vi "nanocal frontend 18.vi"() -> ()   [LabVIEW 2018]
uses:
  nanocal/Nanocalorimetry/data/NanoCalLib.lvlibp/NanoReadings/NanoReadings_Parameters_TypeDef.ctl
  nanocal/Nanocalorimetry/data/NanoCalLib.lvlibp/NanoReadings/NanoReadings_Power.ctl
  nanocal/Nanocalorimetry/data/NanoCalLib.lvlibp/NanoReadings/NanoReadings_CandK.ctl
  nanocal/Nanocalorimetry/data/NanoCalLib.lvlibp/NanoReadings/NanoReadings_IandV.ctl
  nanocal/Nanocalorimetry/data/NanoCalLib.lvlibp/NanoReadings/NanoReadings_TdcTac.ctl
  nanocal/Nanocalorimetry/data/NanoCalLib.lvlibp/NanoReadings/NanoReadings_Phases.ctl
  nanocal/Nanocalorimetry/data/NanoCalLib.lvlibp/NanoReadings/NanoReadings_Frequencies.ctl
  nanocal/Nanocalorimetry/data/NanoCalLib.lvlibp/NanoReadings/NanoReadings_FirstHarmonic.ctl
  nanocal/Nanocalorimetry/data/NanoCalLib.lvlibp/NanoReadings/NanoReadings_Output.ctl
  nanocal/Nanocalorimetry/data/NanoCalLib.lvlibp/NanoReadings/NanoReadings_MagneticFieldEtc.ctl
  nanocal/Nanocalorimetry/data/NanoCalLib.lvlibp/NanoReadings/NanoReadings_Calibration.ctl
  nanocal/Nanocalorimetry/data/NanoCalLib.lvlibp/NanoReadings/NanoReadings_CTetc.ctl
  nanocal/Nanocalorimetry/data/NanoCalLib.lvlibp/NanoReadings/NanoReadings_2ndHarmonic.ctl
  nanocal/Nanocalorimetry/data/NanoCalLib.lvlibp/NanoReadings/NanoReadings_Resistance.ctl
  nanocal/Nanocalorimetry/data/NanoCalLib.lvlibp/NanoReadings/NanoReadings_TimeEtc.ctl
  frontend -- data type -- folder/frontend -- data type.ctl
  nanocal/Nanocalorimetry/data/NanoCalLib.lvlibp
  nanocal/Nanocalorimetry/data/NanoCalLib.lvlibp/NanoReadings/NanoReadings.lvlib
panel:
  out "Numeric":i32=90
  out "output cluster":T1
  in  "milliseconds to wait":u32=100
  in  "Stop":bool
  out "Latest data":T2 {"Time etc"."Datapoint time (s)" format="%#_7g"; "Time etc"."Datapoint index" format="%#_7g"; "Time etc"."Time (s)" format="%#_7g"; "Resistance"."Roffs (ohm)" format="%#_7g"; "Resistance"."Rr,ac (ohm)" format="%#_7g"; "Resistance"."Rs,ac (ohm)" format="%#_7g"; "Resistance"."RHr,dc (ohm)" format="%#_7g"; "Resistance"."RHs,dc (ohm)" format="%#_7g"; "Resistance"."Rr (ohm)" format="%#_7g"; "Resistance"."Rs (ohm)" format="%#_7g"; "Resistance"."RHr (ohm)" format="%#_7g"; "Resistance"."RHs (ohm)" format="%#_7g"; "IV 2nd harm"."Udiff,ac (V)" format="%#_7g"; "IV 2nd harm"."Ur,ac (V)" format="%#_7g"; "IV 2nd harm"."Us,ac (V)" format="%#_7g"; "IV 2nd harm"."Ir,ac (A)" format="%#_7g"; "IV 2nd harm"."Is,ac (A)" format="%#_7g"; "CT etc"."Tr^2 (K^2)" format="%#_7g"; "CT etc"."Ts^2 (K^2)" format="%#_7g"; "Calibration"."dTr/dt (mK/s)" format="%#_7g"; "Calibration"."dTs/dt (mK/s)" format="%#_7g"; "Output"."Hr dc out (V)" min=0.0 max=7.0707; "Output"."Hs dc out (V)" min=0.0 max=7.0707; "Output"."Hr ac out (Vrms)" min=0.0 max=7.0707; "Output"."Hs ac out (Vrms)" min=0.0 max=7.0707; "Output"."R phase (deg)" format="%#_7g"; "Output"."S phase (deg)" format="%#_7g"; "IV 1st harm"."UHr (V)" format="%#_7g"; "IV 1st harm"."IHr (A)" format="%#_7g"; "IV 1st harm"."UHs (V)" format="%#_7g"; "IV 1st harm"."IHs (A)" format="%#_7g"; "IV 1st harm"."Udiff,ac 1st (V)" format="%#_7g"; "IV 1st harm"."Ur,ac 1st (V)" format="%#_7g"; "IV 1st harm"."Us,ac 1st (V)" format="%#_7g"; "IV 1st harm"."Ir,ac 1st (A)" format="%#_7g"; "IV 1st harm"."Is,ac 1st (A)" format="%#_7g"; "f etc"."tau (s)" format="%#_7g"; "f etc"."Cos Phi" format="%#_7g"; "f etc"."Sin Phi" format="%#_7g"; "f etc"."Tan Phi S/diff" format="%#_7g"; "Phases"."Phi Udiff, raw (deg)" format="%#_7g"; "Phases"."Phi Udiff 1st (deg)" format="%#_7g"; "Phases"."Phi Ur 1st (deg)" format="%#_7g"; "Phases"."Phi Ir 1st (deg)" format="%#_7g"; "Phases"."Phi Us 1st (deg)" format="%#_7g"; "Phases"."Phi Is 1st (deg)" format="%#_7g"; "Phases"."Phi R from S,diff (deg)" format="%#_7g"; "Phases"."Phi UHr (deg)" format="%#_7g"; "Phases"."Phi IHr (deg)" format="%#_7g"; "Phases"."Phi UHs (deg)" format="%#_7g"; "Phases"."Phi IHs (deg)" format="%#_7g"; "Phases"."Phi Udiff (deg)" format="%#_7g"; "Phases"."Phi Ur (deg)" format="%#_7g"; "Phases"."Phi Ir (deg)" format="%#_7g"; "Phases"."Phi Us (deg)" format="%#_7g"; "Phases"."Phi Is (deg)" format="%#_7g"; "Tdc,Tac"."T target (K)" format="%#_7g"; "Tdc,Tac"."Tr,ac from Ts,diff,ac (K)" format="%#_7g"; "Tdc,Tac"."Tr,ac driftcorr (K)" format="%#_7g"; "Tdc,Tac"."Ts,ac driftcorr (K)" format="%#_7g"; "Tdc,Tac"."Tdiff,ac (K)" format="%#_7g"; "Tdc,Tac"."Tr,ac (K)" format="%#_7g"; "Tdc,Tac"."Ts,ac (K)" format="%#_7g"; "Tdc,Tac"."Tdiff from Udiff (K)" format="%#_7g"; "Tdc,Tac"."Tdiff from Rs,Rr" format="%#_7g"; "Tdc,Tac"."Tr (K)" format="%#_7g"; "Tdc,Tac"."Ts (K)" format="%#_7g"; "IV dc"."Ioffs dc (A)" format="%#_7g"; "IV dc"."Uoffs dc (V)" format="%#_7g"; "IV dc"."UHr dc (V)" format="%#_7g"; "IV dc"."IHr dc (A)" format="%#_7g"; "IV dc"."UHs dc (V)" format="%#_7g"; "IV dc"."IHs dc (A)" format="%#_7g"; "IV dc"."Udiff,dc (V)" format="%#_7g"; "IV dc"."Ur,dc (V)" format="%#_7g"; "IV dc"."Us,dc (V)" format="%#_7g"; "IV dc"."Ir,dc (A)" format="%#_7g"; "IV dc"."Is,dc (A)" format="%#_7g"; "Power"."Ps,offs (W)" format="%#_7g"; "Power"."Ps-Pr total (W)" format="%#_7g"; "Power"."Pr total (W)" format="%#_7g"; "Power"."Ps total (W)" format="%#_7g"; "Power"."Poffs (W)" format="%#_7g"; "Power"."PHs/PHr" format="%#_7g"; "Power"."Pr,ac (W)" format="%#_7g"; "Power"."Ps,ac (W)" format="%#_7g"; "Power"."PHr,dc (W)" format="%#_7g"; "Power"."PHs,dc (W)" format="%#_7g"; "Power"."Pr,dc (W)" format="%#_7g"; "Power"."Ps,dc (W)" format="%#_7g"; "Power"."PHr (W)" format="%#_7g"; "Power"."PHs (W)" format="%#_7g"}
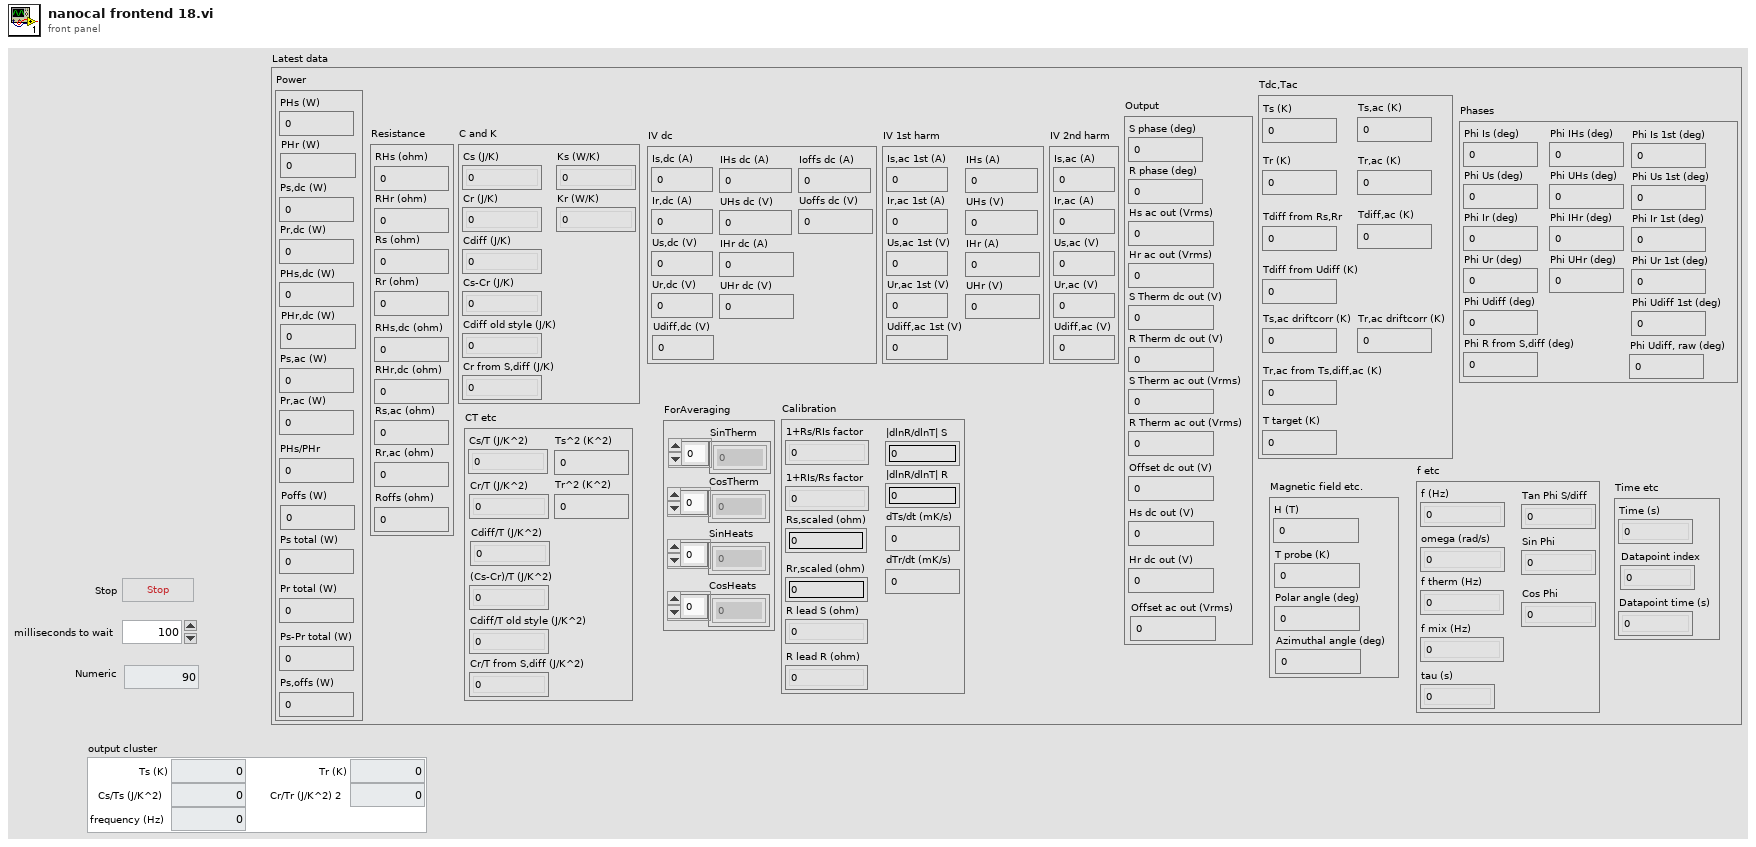
[diagram p1: front panel]
types:
  T1 = typedef "frontend -- data type.ctl" = cluster{"frequency (Hz)":dbl, "Cs/Ts (J/K^2)":dbl, "Ts (K)":dbl, "Cr/Tr (J/K^2) 2":dbl, "Tr (K)":dbl}
  T2 = typedef "NanoCalLib.lvlibp/NanoReadings.lvlib/NanoReadings_Parameters_TypeDef.ctl" = cluster{"Power":T3, "C and K":T4, "IV dc":T5, "Tdc,Tac":T6, "Phases":T7, "f etc":T8, "IV 1st harm":T9, "ForAveraging":cluster{"SinTherm":dbl[], "CosTherm":dbl[], "SinHeats":dbl[], "CosHeats":dbl[]}, "Output":T10, "Magnetic field etc.":T11, "Calibration":T12, "CT etc":T13, "IV 2nd harm":T14, "Resistance":T15, "Time etc":T16}
  T3 = typedef "NanoCalLib.lvlibp/NanoReadings.lvlib/NanoReadings_Power.ctl" = cluster{"PHs (W)":dbl, "PHr (W)":dbl, "Ps,dc (W)":dbl, "Pr,dc (W)":dbl, "PHs,dc (W)":dbl, "PHr,dc (W)":dbl, "Ps,ac (W)":dbl, "Pr,ac (W)":dbl, "PHs/PHr":dbl, "Poffs (W)":dbl, "Ps total (W)":dbl, "Pr total (W)":dbl, "Ps-Pr total (W)":dbl, "Ps,offs (W)":dbl}
  T4 = typedef "NanoCalLib.lvlibp/NanoReadings.lvlib/NanoReadings_CandK.ctl" = cluster{"Cs (J/K)":dbl, "Ks (W/K)":dbl, "Cr (J/K)":dbl, "Kr (W/K)":dbl, "Cdiff (J/K)":dbl, "Cs-Cr (J/K)":dbl, "Cdiff old style (J/K)":dbl, "Cr from S,diff (J/K)":dbl}
  T5 = typedef "NanoCalLib.lvlibp/NanoReadings.lvlib/NanoReadings_IandV.ctl" = cluster{"Is,dc (A)":dbl, "Ir,dc (A)":dbl, "Us,dc (V)":dbl, "Ur,dc (V)":dbl, "Udiff,dc (V)":dbl, "IHs dc (A)":dbl, "UHs dc (V)":dbl, "IHr dc (A)":dbl, "UHr dc (V)":dbl, "Uoffs dc (V)":dbl, "Ioffs dc (A)":dbl}
  T6 = typedef "NanoCalLib.lvlibp/NanoReadings.lvlib/NanoReadings_TdcTac.ctl" = cluster{"Ts (K)":dbl, "Tr (K)":dbl, "Tdiff from Rs,Rr":dbl, "Tdiff from Udiff (K)":dbl, "Ts,ac (K)":dbl, "Tr,ac (K)":dbl, "Tdiff,ac (K)":dbl, "Ts,ac driftcorr (K)":dbl, "Tr,ac driftcorr (K)":dbl, "Tr,ac from Ts,diff,ac (K)":dbl, "T target (K)":dbl}
  T7 = typedef "NanoCalLib.lvlibp/NanoReadings.lvlib/NanoReadings_Phases.ctl" = cluster{"Phi Is (deg)":dbl, "Phi Us (deg)":dbl, "Phi Ir (deg)":dbl, "Phi Ur (deg)":dbl, "Phi Udiff (deg)":dbl, "Phi IHs (deg)":dbl, "Phi UHs (deg)":dbl, "Phi IHr (deg)":dbl, "Phi UHr (deg)":dbl, "Phi R from S,diff (deg)":dbl, "Phi Is 1st (deg)":dbl, "Phi Us 1st (deg)":dbl, "Phi Ir 1st (deg)":dbl, "Phi Ur 1st (deg)":dbl, "Phi Udiff 1st (deg)":dbl, "Phi Udiff, raw (deg)":dbl}
  T8 = typedef "NanoCalLib.lvlibp/NanoReadings.lvlib/NanoReadings_Frequencies.ctl" = cluster{"f (Hz)":dbl, "f therm (Hz)":dbl, "omega (rad/s)":dbl, "Tan Phi S/diff":dbl, "Sin Phi":dbl, "Cos Phi":dbl, "f mix (Hz)":dbl, "tau (s)":dbl}
  T9 = typedef "NanoCalLib.lvlibp/NanoReadings.lvlib/NanoReadings_FirstHarmonic.ctl" = cluster{"Is,ac 1st (A)":dbl, "Ir,ac 1st (A)":dbl, "Us,ac 1st (V)":dbl, "Ur,ac 1st (V)":dbl, "Udiff,ac 1st (V)":dbl, "IHs (A)":dbl, "UHs (V)":dbl, "IHr (A)":dbl, "UHr (V)":dbl}
  T10 = typedef "NanoCalLib.lvlibp/NanoReadings.lvlib/NanoReadings_Output.ctl" = cluster{"S phase (deg)":dbl, "R phase (deg)":dbl, "Hs ac out (Vrms)":dbl, "Hr ac out (Vrms)":dbl, "S Therm dc out (V)":dbl, "R Therm dc out (V)":dbl, "S Therm ac out (Vrms)":dbl, "R Therm ac out (Vrms)":dbl, "Offset dc out (V)":dbl, "Hs dc out (V)":dbl, "Hr dc out (V)":dbl, "Offset ac out (Vrms)":dbl}
  T11 = typedef "NanoCalLib.lvlibp/NanoReadings.lvlib/NanoReadings_MagneticFieldEtc.ctl" = cluster{"H (T)":dbl, "T probe (K)":dbl, "Polar angle (deg)":dbl, "Azimuthal angle (deg)":dbl}
  T12 = typedef "NanoCalLib.lvlibp/NanoReadings.lvlib/NanoReadings_Calibration.ctl" = cluster{"1+Rs/RIs factor":dbl, "1+RIs/Rs factor":dbl, "Rs,scaled (ohm)":dbl, "Rr,scaled (ohm)":dbl, "R lead S (ohm)":dbl, "R lead R (ohm)":dbl, "|dlnR/dlnT| S":dbl, "|dlnR/dlnT| R":dbl, "dTs/dt (mK/s)":dbl, "dTr/dt (mK/s)":dbl}
  T13 = typedef "NanoCalLib.lvlibp/NanoReadings.lvlib/NanoReadings_CTetc.ctl" = cluster{"Cs/T (J/K^2)":dbl, "Cr/T (J/K^2)":dbl, "Cdiff/T (J/K^2)":dbl, "(Cs-Cr)/T (J/K^2)":dbl, "Cdiff/T old style (J/K^2)":dbl, "Cr/T from S,diff (J/K^2)":dbl, "Ts^2 (K^2)":dbl, "Tr^2 (K^2)":dbl}
  T14 = typedef "NanoCalLib.lvlibp/NanoReadings.lvlib/NanoReadings_2ndHarmonic.ctl" = cluster{"Is,ac (A)":dbl, "Ir,ac (A)":dbl, "Us,ac (V)":dbl, "Ur,ac (V)":dbl, "Udiff,ac (V)":dbl}
  T15 = typedef "NanoCalLib.lvlibp/NanoReadings.lvlib/NanoReadings_Resistance.ctl" = cluster{"RHs (ohm)":dbl, "RHr (ohm)":dbl, "Rs (ohm)":dbl, "Rr (ohm)":dbl, "RHs,dc (ohm)":dbl, "RHr,dc (ohm)":dbl, "Rs,ac (ohm)":dbl, "Rr,ac (ohm)":dbl, "Roffs (ohm)":dbl}
  T16 = typedef "NanoCalLib.lvlibp/NanoReadings.lvlib/NanoReadings_TimeEtc.ctl" = cluster{"Time (s)":dbl, "Datapoint index":dbl, "Datapoint time (s)":dbl}
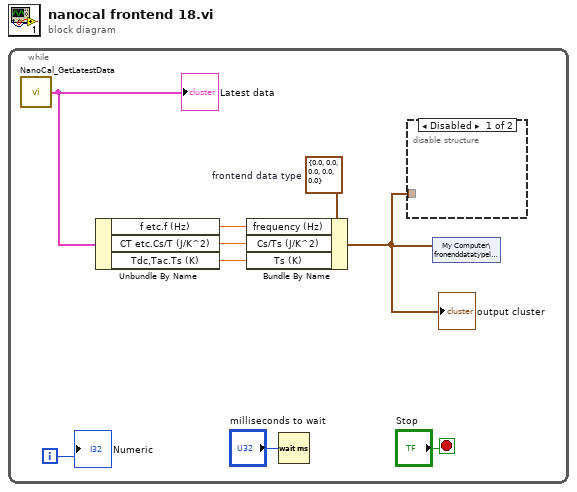
[diagram p0: block diagram]
diagram:
  n1 = while {
    i -> [w4]
    stop <- "Stop" stop-if-true
    w7 = T1 {"frequency (Hz)"=0.0, "Cs/Ts (J/K^2)"=0.0, "Ts (K)"=0.0, "Cr/Tr (J/K^2) 2"=0.0, "Tr (K)"=0.0}  # frontend data type
    n2 = call "NanoCal_GetLatestData.vi"() -> ("Latest data"=w3:T2)  [unwired: 1 in]
    "Latest data" <- w3
    n3 = Unbundle By Name(w3) -> ("f etc.f (Hz)"=w6:dbl, "CT etc.Cs/T (J/K^2)"=w5:dbl, "Tdc,Tac.Ts (K)"=w2:dbl)
    n4 = Bundle By Name(cluster=w7, "frequency (Hz)"=w6, "Cs/Ts (J/K^2)"=w5, "Ts (K)"=w2) -> (w1:T1)
    "output cluster" <- w1
    n5 = Wait (ms)(milliseconds to wait="milliseconds to wait") -> ()  [unwired: 1 out]
    n6 = disable-structure shown="Disabled" {
      disable-tunnel: w1 -> [_ _]
      frame Disabled {
      }
      frame Enabled {
      }
    }
    n7 = shared-variable "My Computer\\fronenddatatypelib.lvlib\\data"(w1) -> ()  [unwired: 1 in, 1 out]
    "Numeric" <- w4
  }
